vi "for_v0_v20.vi"() -> ()   [LabVIEW 2009]
panel:
  in  "stop":bool
  out "Graficul functiei e^x":dbl[](graph)=[1.0, 2.718281828459045, 7.38905609893065, 20.085536923187668, 54.598150033144236, 148.4131591025766, 403.4287934927351, 1096.6331584284585, 2980.9579870417283]
  in  "Numar dde puncte":u8(slide)=9 scale=0.0..20.0
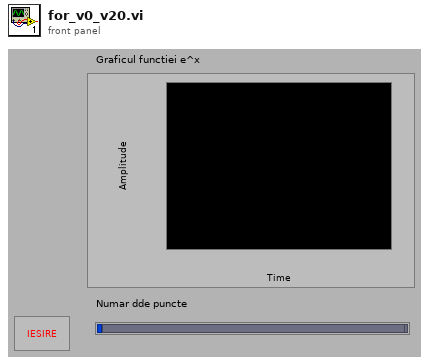
[diagram p1: front panel]
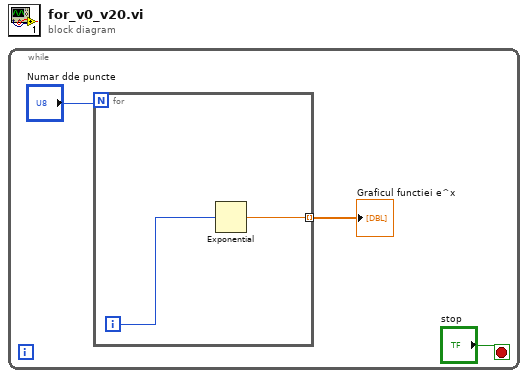
[diagram p0: block diagram]
diagram:
  n1 = while {
    stop <- "stop" stop-if-true
    n2 = for {
      N: "Numar dde puncte" -> [_]
      tunnel: [w5] -> w3 mode=indexing
      i -> [w4]
      n3 = Exponential(1:w4) -> (0:w5:dbl)
    }
    "Graficul functiei e^x" <- w3
  }
